vi "Begin.vi"() -> (0 "error out":errorcluster)   [LabVIEW 2014]
doc: "Called before other user functions, this VI is expected to open initial I/O refnums, load in file data, and do all program initialization. Notice that the <B>error out</B> terminal is simply used for data flow. Wiring it to other structures or subVIs ensures that this VI runs first."
uses:
  <vilib>/Rock Robotics/WPI/DriverStation/WPI_DriverStationRobotMode2.ctl
  <vilib>/Rock Robotics/SystemInterfaces/Typedef/FPGA_TypedefAnalogModule.ctl
  <vilib>/Rock Robotics/SystemInterfaces/AI/FPGA_AIChannel.ctl
  <vilib>/Rock Robotics/WPI/Joystick/WPI_JoystickDeviceEnum.ctl
  Robot Global Data.vi
  navX-MXP-LabVIEW/navX-MXP Library/navX-MXP IMU.lvlib
panel:
  in  "Ramp Rate":dbl=50.0
  in  "Extension PID":cluster{"P":dbl, "I":dbl, "D":dbl}
  in  "Wrist  PID":cluster{"P":dbl, "I":dbl, "D":dbl}
  in  "Pivot PID":cluster{"P":dbl, "I":dbl, "D":dbl}
  in  "Speed PID":cluster{"P":dbl, "I":dbl, "D":dbl}={"P"=0.0275, "I"=0.000115, "D"=0.682955}
  in  "Steering PID":cluster{"P":dbl, "I":dbl, "D":dbl}={"P"=48.0, "I"=0.0, "D"=638.0}
  in  "error in":errorcluster
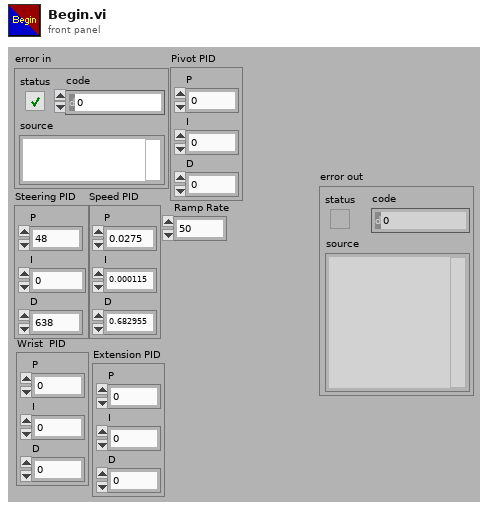
[diagram p1: front panel]
types:
  T1 = typedef "WPI_DriverStationRobotMode2.ctl" = enum16{"Autonomous Disabled", "Autonomous Enabled", "Teleop Disabled", "Teleop Enabled", "Disconnected", "Finish", "Test Disabled", "Test Enabled", "Emergency Stopped"}
  T2 = typedef "FPGA_AIChannel.ctl" = enum8{"AI 0", "AI 1", "AI 2", "AI 3", "AI MXP 0", "AI MXP 1", "AI MXP 2", "AI MXP 3", "Invalid"}
  T3 = typedef "FPGA_TypedefAnalogModule.ctl" = enum16{"Controller 1"}
  T4 = typedef "WPI_AnalogChannelDevRef.ctl" = cluster{"DevStatus":errorcluster, "Controller":T3, "Analog Channel":T2}
  T5 = typedef "navX-MXP IMU.lvlib/navX Device TypeDef.ctl" = cluster{"navX Interface Protocol":T6, "navX Interface Protocol TypeDefs":cluster{"SPIDevRef":T7, "I2CDevRef":T10}, "navX System Information":cluster{"Board Information":T12, "Status":T13, "Offsets":T17}, "navX Common Information":cluster{"Update Rate (4Hz-60Hz)":T18, "refnum name":string, "error":errorcluster}}
  T6 = typedef "navX-MXP IMU.lvlib/navX Interface Protocol.ctl" = enum16{"SPI", "I2C"}
  T7 = typedef "WPI_SPIDevRef.ctl" = cluster{"DevStatus":errorcluster, "Handle":i32, "Controller":T8, "SPI Bus":T9}
  T8 = typedef "FPGA_TypedefDigitalModule.ctl" = enum16{"Controller 1"}
  T9 = typedef "spi_bus.ctl" = enum16{"SPI On-Board, CS0", "SPI On-Board, CS1", "SPI On-Board, CS2", "SPI On-Board, CS3", "SPI MXP", "Invalid"}
  T10 = typedef "WPI_I2CDevRef.ctl" = cluster{"DevStatus":errorcluster, "Controller":T8, "Device Address":u8, "Handle":i32, "I2C Bus":T11}
  T11 = typedef "i2c_bus.ctl" = enum16{"I2C On-Board", "I2C MXP", "Invalid"}
  T12 = typedef "navX-MXP IMU.lvlib/navX Board Information.ctl" = cluster{"WhoAmI (50 | 0x32)":u8, "Board Revision":u8, "Firmware Major Version":u8, "Firmware Minor Version":u8}
  T13 = typedef "navX-MXP IMU.lvlib/navX Status Data.ctl" = cluster{"Update Rate Hz":u8, "Accelerometer Full-Scale Range":u8, "Gyro Full-Scale Range":u16, "NAVX_OP_STATUS":T14, "NAVX_CAL_STATUS":T15, "NAVX_SELFTEST_STATUS":u8, "NAVX_SENSOR_STATUS":T16}
  T14 = typedef "navX-MXP IMU.lvlib/navX NAVX_OP_STATUS.ctl" = u8
  T15 = typedef "navX-MXP IMU.lvlib/navX NAVX_CAL_STATUS.ctl" = u8
  T16 = typedef "navX-MXP IMU.lvlib/navX NAVX_SENSOR_STATUS.ctl" = cluster{"MOVING":bool, "YAW_STABLE":bool, "MAG_DISTURBANCE":bool, "ALTITUDE_VALID":bool, "SEALEVEL_PRESS_SET":bool, "FUSED_HEADING_VALID":bool}
  T17 = typedef "navX-MXP IMU.lvlib/navX Offsets Data.ctl" = cluster{"Yaw":dbl, "Quat W":dbl, "Quat X":dbl, "Quat Y":dbl, "Quat Z":dbl}
  T18 = typedef "navX-MXP IMU.lvlib/navX Update Rate.ctl" = u8
  T19 = typedef "WPI_JoystickDeviceEnum.ctl" = enum16{"USB 0", "USB 1", "USB 2", "USB 3", "USB 4", "USB 5"}
  T20 = typedef "WPI_JoystickDevRef.ctl" = cluster{"Device":T19}
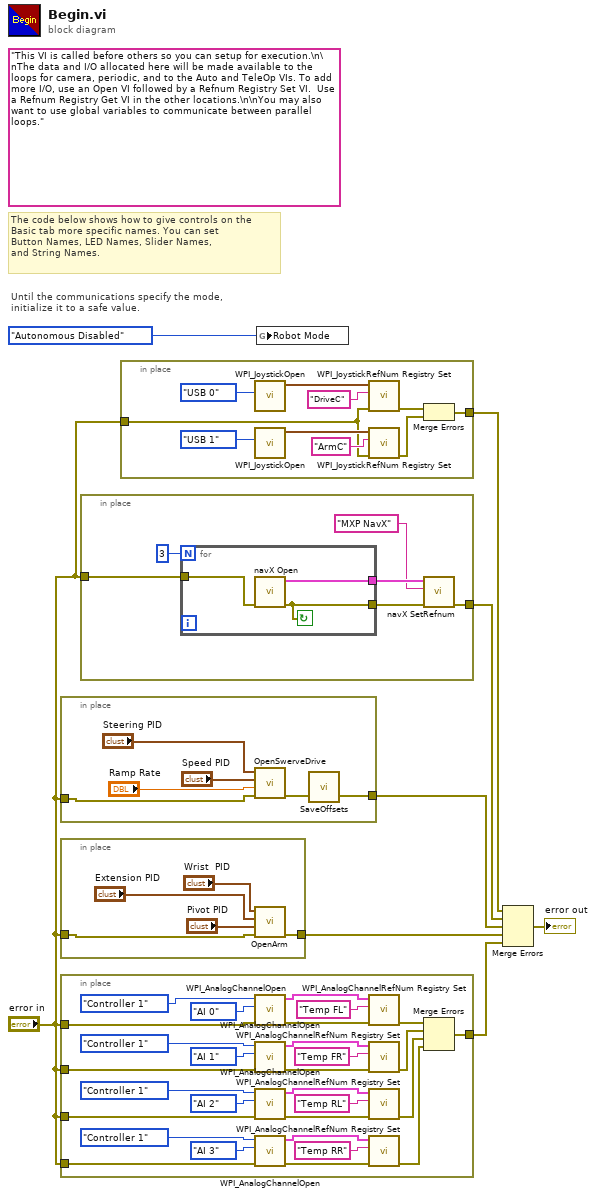
[diagram p0: block diagram]
diagram:
  (unwired) "This VI is called before others so you can setup for execution.\n\nThe data and I/O allocated here will be made available to the loops for camera, periodic, and to the Auto and TeleOp VIs. To add more I/O, use an Open VI followed by a Refnum Registry Set VI.  Use a Refnum Registry Get VI in the other locations.\n\nYou may also want to use global variables to communicate between parallel loops."
  # "The code below shows how to give controls on the\nBasic tab more specific names. You can set\nButton Names, LED Names, Slider Names,\nand String Names."
  # "Until the communications specify the mode,\ninitialize it to a safe value."
  n1 = in-place {
    in-place-border: [w9] -> w4
    in-place-border: "error in" -> [w14]
    n2 = call "OpenSwerveDrive.vi"("error in"=w14, "Ramp Rate"="Ramp Rate", "Speed PID"="Speed PID", "Steering PID"="Steering PID") -> ("error out"=w10:errorcluster)  [unwired: 5 in]
    n3 = call "SaveOffsets.vi"("error in"=w10) -> ("error out"=w9:errorcluster)  [unwired: 2 in]
  }
  n4 = in-place {
    in-place-border: [w19] -> w3
    in-place-border: "error in" -> [w18]
    n5 = call "OpenArm.vi"("error in (no error)"=w18, "Pivot PID"="Pivot PID", "Extension PID"="Extension PID", "Wrist  PID"="Wrist  PID") -> ("error out"=w19:errorcluster)  [unwired: 7 in]
  }
  n6 = in-place {
    in-place-border: "error in" -> [w48]
    in-place-border: "error in" -> [w47]
    in-place-border: "error in" -> [w46]
    in-place-border: "error in" -> [w45]
    in-place-border: [w44] -> w1
    n7 = call <vilib>:"WPI_AnalogChannelOpen.vi"("error in (no error)"=w48, "Analog Channel"=FPGA_AIChannel."AI 0", "Controller"=FPGA_TypedefAnalogModule."Controller 1") -> ("error out"=w32:errorcluster, "AIDeviceRef"=w25:T4)  [unwired: 7 in]
    n8 = call <vilib>:"WPI_AnalogChannelOpen.vi"("error in (no error)"=w47, "Analog Channel"=FPGA_AIChannel."AI 1", "Controller"=FPGA_TypedefAnalogModule."Controller 1") -> ("error out"=w34:errorcluster, "AIDeviceRef"=w35:T4)  [unwired: 7 in]
    n9 = call <vilib>:"WPI_AnalogChannelOpen.vi"("error in (no error)"=w45, "Analog Channel"=FPGA_AIChannel."AI 2", "Controller"=FPGA_TypedefAnalogModule."Controller 1") -> ("error out"=w26:errorcluster, "AIDeviceRef"=w23:T4)  [unwired: 7 in]
    n10 = call <vilib>:"WPI_AnalogChannelOpen.vi"("error in (no error)"=w46, "Analog Channel"=FPGA_AIChannel."AI 3", "Controller"=FPGA_TypedefAnalogModule."Controller 1") -> ("error out"=w27:errorcluster, "AIDeviceRef"=w22:T4)  [unwired: 7 in]
    n11 = call <vilib>:"WPI_AnalogChannelRefNum Registry Set.vi"("error in (no error)"=w32, "refnum name"="Temp FL", "AIDeviceRef"=w25) -> ("error out"=w31:errorcluster)  [unwired: 7 in, 1 out]
    n12 = call <vilib>:"WPI_AnalogChannelRefNum Registry Set.vi"("error in (no error)"=w34, "refnum name"="Temp FR", "AIDeviceRef"=w35) -> ("error out"=w30:errorcluster)  [unwired: 7 in, 1 out]
    n13 = call <vilib>:"WPI_AnalogChannelRefNum Registry Set.vi"("error in (no error)"=w26, "refnum name"="Temp RL", "AIDeviceRef"=w23) -> ("error out"=w29:errorcluster)  [unwired: 7 in, 1 out]
    n14 = call <vilib>:"WPI_AnalogChannelRefNum Registry Set.vi"("error in (no error)"=w27, "refnum name"="Temp RR", "AIDeviceRef"=w22) -> ("error out"=w28:errorcluster)  [unwired: 7 in, 1 out]
    n15 = Merge Errors(w31, w30, w29, w28) -> (w44:errorcluster)
  }
  n16 = in-place {
    in-place-border: [w54] -> w5
    in-place-border: "error in" -> [w51]
    n17 = for {
      N: 3 -> [_]
      tunnel: [w57] -> w52
      tunnel: w51 -> [w56]
      tunnel: [w55] -> w53
      stop <- w55 continue-if-true
      n18 = call "navX Open.vi"("error in"=w56) -> ("error out"=w55:errorcluster, "navX Device TypeDef"=w57:T5)  [unwired: 8 in, 1 out]
    }
    n19 = call "navX SetRefnum.vi"("error in (no error)"=w53, "refnum name"="MXP NavX", "navX Device TypeDef"=w52) -> ("error out"=w54:errorcluster)  [unwired: 7 in, 1 out]
  }
  n20 = in-place {
    in-place-border: [w59] -> w6
    in-place-border: "error in" -> [w60]
    n21 = call <vilib>:"WPI_JoystickOpen.vi"("JoystickDevice"=WPI_JoystickDeviceEnum."USB 0") -> ("JoystickDevRef"=w66:T20)  [unwired: 10 in]
    n22 = call <vilib>:"WPI_JoystickOpen.vi"("JoystickDevice"=WPI_JoystickDeviceEnum."USB 1") -> ("JoystickDevRef"=w63:T20)  [unwired: 10 in]
    n23 = call <vilib>:"WPI_JoystickRefNum Registry Set.vi"("error in (no error)"=w60, "refnum name"="DriveC", "JoystickDevRef"=w66) -> ("error out"=w67:errorcluster)  [unwired: 7 in, 1 out]
    n24 = call <vilib>:"WPI_JoystickRefNum Registry Set.vi"("error in (no error)"=w60, "refnum name"="ArmC", "JoystickDevRef"=w63) -> ("error out"=w58:errorcluster)  [unwired: 7 in, 1 out]
    n25 = Merge Errors(w67, w58) -> (w59:errorcluster)
  }
  n26 = global write "Robot Global Data.vi" "Robot Mode"(WPI_DriverStationRobotMode2."Autonomous Disabled" ("Robot Mode")) -> ()
  n27 = Merge Errors(w6, w5, w4, w3, w1) -> (→"error out":errorcluster)
